vi "JSON to Schemes.vi"(11 "Material JSON":string) -> (0 "error out":errorcluster, 3 "Schemes":refnum<class "Material-Scheme.lvclass">[](array[class]))   [LabVIEW 2021, in "TSC Material Theme.lvlib" / "Material-Scheme.lvclass"]
uses:
  Material-Scheme.lvclass
  Serializer-Scheme/Serializer-Scheme.lvclass
  <vilib>/JDP Science/JSONtext/JSONtext.lvlib
  bcc1f051-5bb6-434e-b816-a57df783be2e.vi
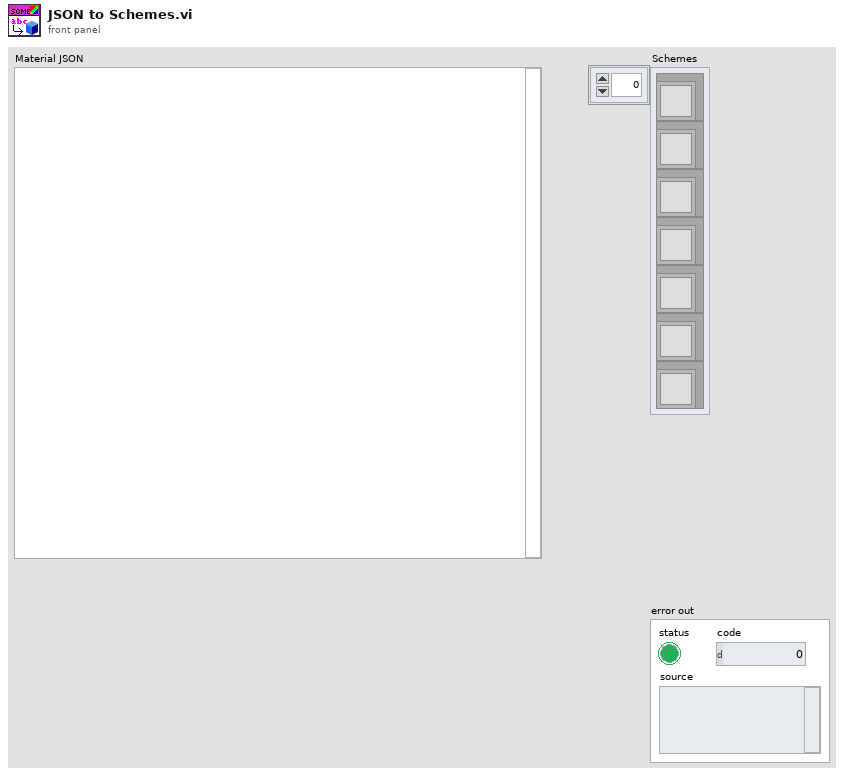
[diagram p1: front panel]
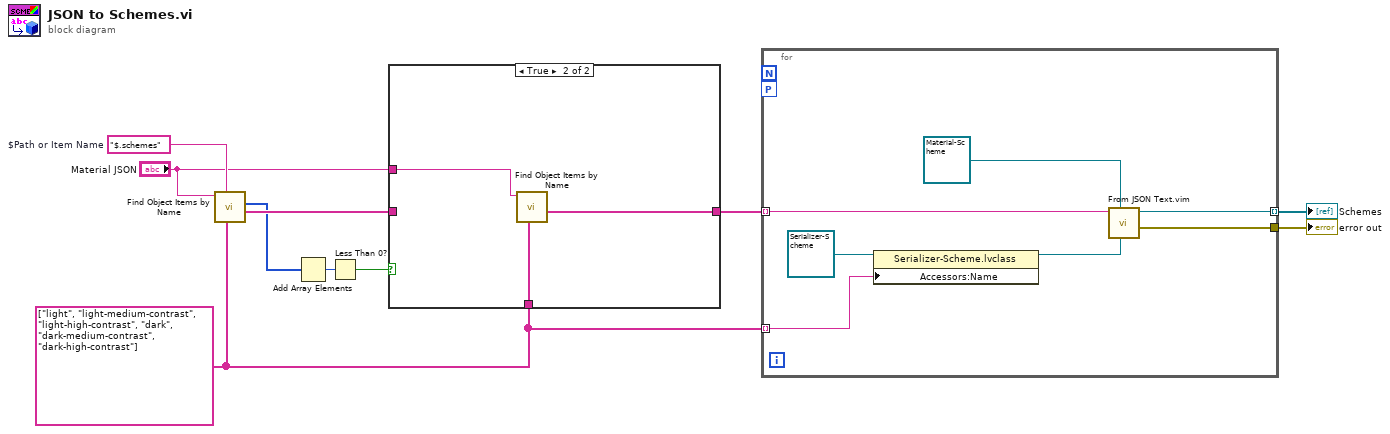
[diagram p0: block diagram]
diagram:
  w9 = "$.schemes"  # $Path or Item Name
  w5 = string[] ["light", "light-medium-contrast", "light-high-contrast", "dark", "dark-medium-contrast", "dark-high-contrast"] ("Item Names")
  n1 = call <vilib>:"Find Object Items by Name.vi"("Item Names"=w5, "$Path or Item Name"=w9, "JSON"="Material JSON") -> ("<JSON>"=w7:string[], "Offsets"=w3:i32[])  [unwired: 6 in, 1 out]
  n2 = Add Array Elements(numeric array=w3) -> (sum=w2:i32)
  n3 = Less Than 0?(x=w2) -> (x < 0?=w1:bool)
  n4 = case shown="True" w1 {
    tunnel: w7 -> [w11 _]
    tunnel: [w11 w12] -> w4
    tunnel: "Material JSON" -> [_ w14]
    tunnel: w5 -> [_ w13]
    frame False {
    }
    frame True {
      n5 = call <vilib>:"Find Object Items by Name.vi"("Item Names"=w13, "JSON"=w14) -> ("<JSON>"=w12:string[])  [unwired: 7 in, 2 out]
    }
  }
  n6 = for {
    tunnel: [w19] -> w8 mode=indexing
    tunnel: [w21] -> w10
    tunnel: w4 -> [w18] mode=indexing
    tunnel: w5 -> [w15] mode=indexing
    workers-P: _ -> [_]
    n7 = property class="Serializer-Scheme.lvclass"(reference=refnum<class "Serializer-Scheme.lvclass"> refnum ("TSC Material Theme.lvlib:Class 1.lvclass"), "Accessors:Name"=w15) -> (reference out=w16:refnum<class "Serializer-Scheme.lvclass">)  [unwired: 1 in, 1 out]
    n8 = call "From JSON Text.vim"("LVClass Serializer"=w16, "Data Type and Default Value"=refnum<class "Material-Scheme.lvclass"> refnum ("TSC Material Theme.lvlib:Material-Scheme"), "JSON"=w18) -> ("error out"=w21:errorcluster, "Data out"=w19:refnum<class "Material-Scheme.lvclass">)  [unwired: 7 in]
  }
  "Schemes" <- w8
  "error out" <- w10
